vi "write TBM configuration.vi"(8 "error in":errorcluster, 10 "configuration":refnum<class "TBM configuration.lvclass">, 11 "Standard Engine Editor Node in":refnum<class "Standard Engine Editor Node.lvclass">) -> (0 "error out":errorcluster, 3 "Standard Engine Editor Node out":refnum<class "Standard Engine Editor Node.lvclass">)   [LabVIEW 2013, in "Standard Engine Editor Node.lvclass"]
uses:
  Standard Engine Editor Node.lvclass
  <vilib>/NI/TBM Engines/Standard Engine/Configuration/Standard Engine Configuration.lvclass
  <vilib>/NI/Tag Bus Module Framework/root configuration/TBM configuration.lvclass
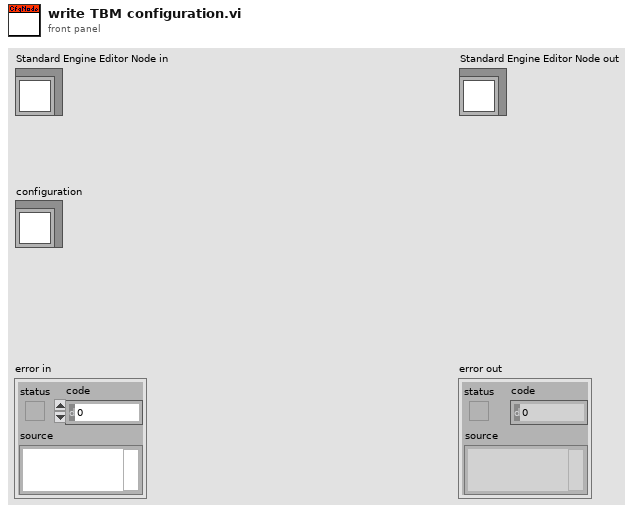
[diagram p1: front panel]
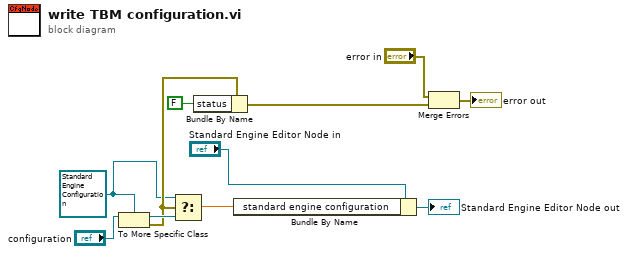
[diagram p0: block diagram]
diagram:
  w5 = refnum<class "Standard Engine Configuration.lvclass"> refnum ("standard engine configuration")
  n1 = To More Specific Class(target class=w5, reference="configuration") -> (specific class reference=w11:refnum<class "Standard Engine Configuration.lvclass">, error out=w10:errorcluster)  [unwired: 1 in]
  n2 = Select(t=w5, s=w10, f=w11) -> (s? t:f=w7:dbl)
  n3 = Bundle By Name(cluster=w10, "status"=FALSE) -> (w8:errorcluster)
  n4 = Bundle By Name(cluster="Standard Engine Editor Node in", "standard engine configuration"=w7) -> (→"Standard Engine Editor Node out":refnum<class "Standard Engine Editor Node.lvclass">)
  n5 = Merge Errors("error in", w8) -> (→"error out":errorcluster)
